vi "Set Dev Stream.vi"(8 "error in (no error)":errorcluster, 9 "firmware revision":string(combo), 10 "dev stream (NORMAL)":u16(ring) items=["NORMAL", "ERROR"], 11 "VISA resource name":refnum<visa-resource-name>) -> (0 "error out":errorcluster, 2 "bridge error":T1, 3 "VISA resource name out":refnum<visa-resource-name>)   [LabVIEW 2019, in "Andeen-Hagerling 2700A.lvlib"]
doc: "Selects whether the E (Error) or the N (Normal) Data Stream will \nsupply the results reported to the front panel and remote devices\nas the result of executing the SINGLE, CONTINUOUS, or FETCH \ncommands while in the deviation mode."
uses:
  Andeen-Hagerling 2700A.lvlib
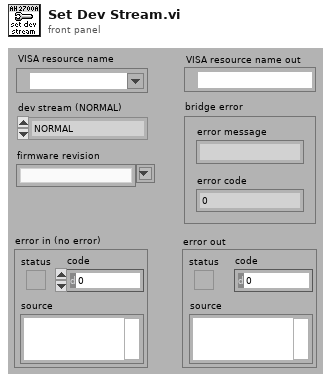
[diagram p1: front panel]
types:
  T1 = cluster{"error message":string, "error code":i32}
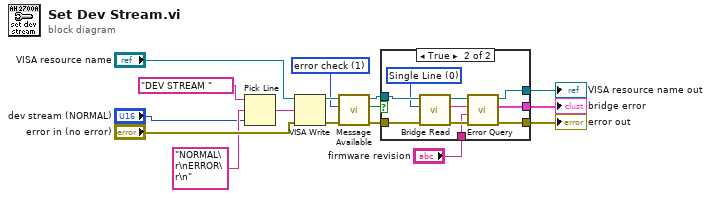
[diagram p0: block diagram]
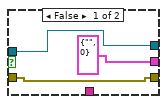
[diagram p2: hidden frame]
diagram:
  w1 = u16 1 items=["none", "error check", "multiline read", "infinite"] ("delay")
  n1 = Pick Line(string ("")="DEV STREAM " ("command"), multi-line string="NORMAL\r\nERROR\r\n" ("options"), line index="dev stream (NORMAL)") -> (output string=w12:string)
  n2 = VISA Write(VISA resource name="VISA resource name", write buffer=w12, error in (no error)="error in (no error)") -> (VISA resource name out=w6:refnum<visa-resource-name>, error out=w5:errorcluster)  [unwired: 1 out]
  n3 = call "Message Available.vi"("error in (no error)"=w5, "delay"=w1, "VISA resource name"=w6) -> ("error out"=w8:errorcluster, "message available"=w10:bool, "VISA resource name out"=w9:refnum<visa-resource-name>)  [unwired: 6 in]
  n4 = case shown="True" w10 {
    tunnel: w9 -> [w18 w26]
    tunnel: w8 -> [w19 w25]
    tunnel: "firmware revision" -> [_ w24]
    tunnel: [w19 w23] -> w3
    tunnel: [w18 w22] -> w4
    tunnel: [T1 {"error message"="", "error code"=0} ("bridge error") w21] -> w2
    frame False {
    }
    frame True {
      w20 = u16 0 items=["Single Line", "Multi-Line"] ("Multiline")
      n5 = call "Bridge Read.vi"("error in (no error)"=w25, "multiline"=w20, "VISA resource name"=w26) -> ("error out"=w28:errorcluster, "read buffer"=w29:string, "VISA resource name out"=w27:refnum<visa-resource-name>)  [unwired: 6 in]
      n6 = call "Error Query.vi"("error in (no error)"=w28, "firmware revision"=w24, "measurement line"=w29, "VISA resource name"=w27) -> ("error out"=w23:errorcluster, "bridge error"=w21:T1, "VISA resource name out"=w22:refnum<visa-resource-name>)  [unwired: 5 in]
    }
  }
  "VISA resource name out" <- w4
  "error out" <- w3
  "bridge error" <- w2
